vi "SelectorTallestTarget.vi"(0 "Array":T1(array[cluster])) -> (7 "VisionClusterOut":T2={"Position"={"Y"=0.0}, "NoTarget"=TRUE, "Right"=TRUE, "Center"=FALSE, "Left"=TRUE, "TargetCenter"=0.0})   [LabVIEW 2011]
panel:
  out "BetterDistanceV2 - Avg":dbl
  out "BetterDistanceMiddle":dbl
  out "BetterDistanceV1":dbl
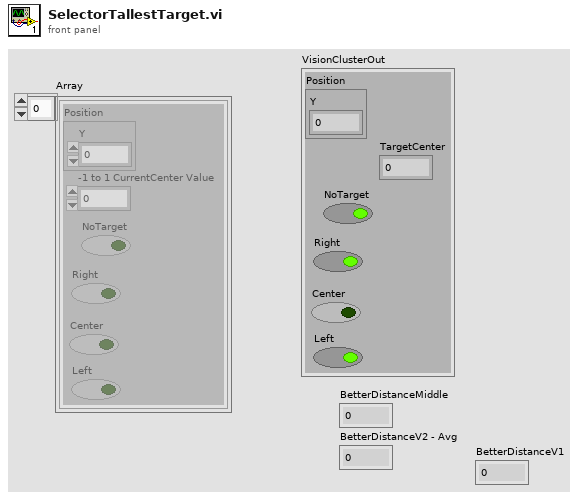
[diagram p1: front panel]
types:
  T1 = cluster{"Position":cluster{"Y":dbl}, "NoTarget":bool, "Right":bool, "Center":bool, "Left":bool, "-1 to 1 CurrentCenter Value":dbl}[]
  T2 = cluster{"Position":cluster{"Y":dbl}, "NoTarget":bool, "Right":bool, "Center":bool, "Left":bool, "TargetCenter":dbl}
  T3 = cluster{"Position":cluster{"X":dbl, "Y":dbl}, "Distance (ft)":dbl, "NoTarget":bool, "Right":bool, "Center":bool, "Left":bool, "TargetCenter":dbl}[]
  T4 = cluster{"Position":cluster{"Y":dbl}, "NoTarget":bool, "Right":bool, "Center":bool, "Left":bool, "-1 to 1 CurrentCenter Value":dbl}
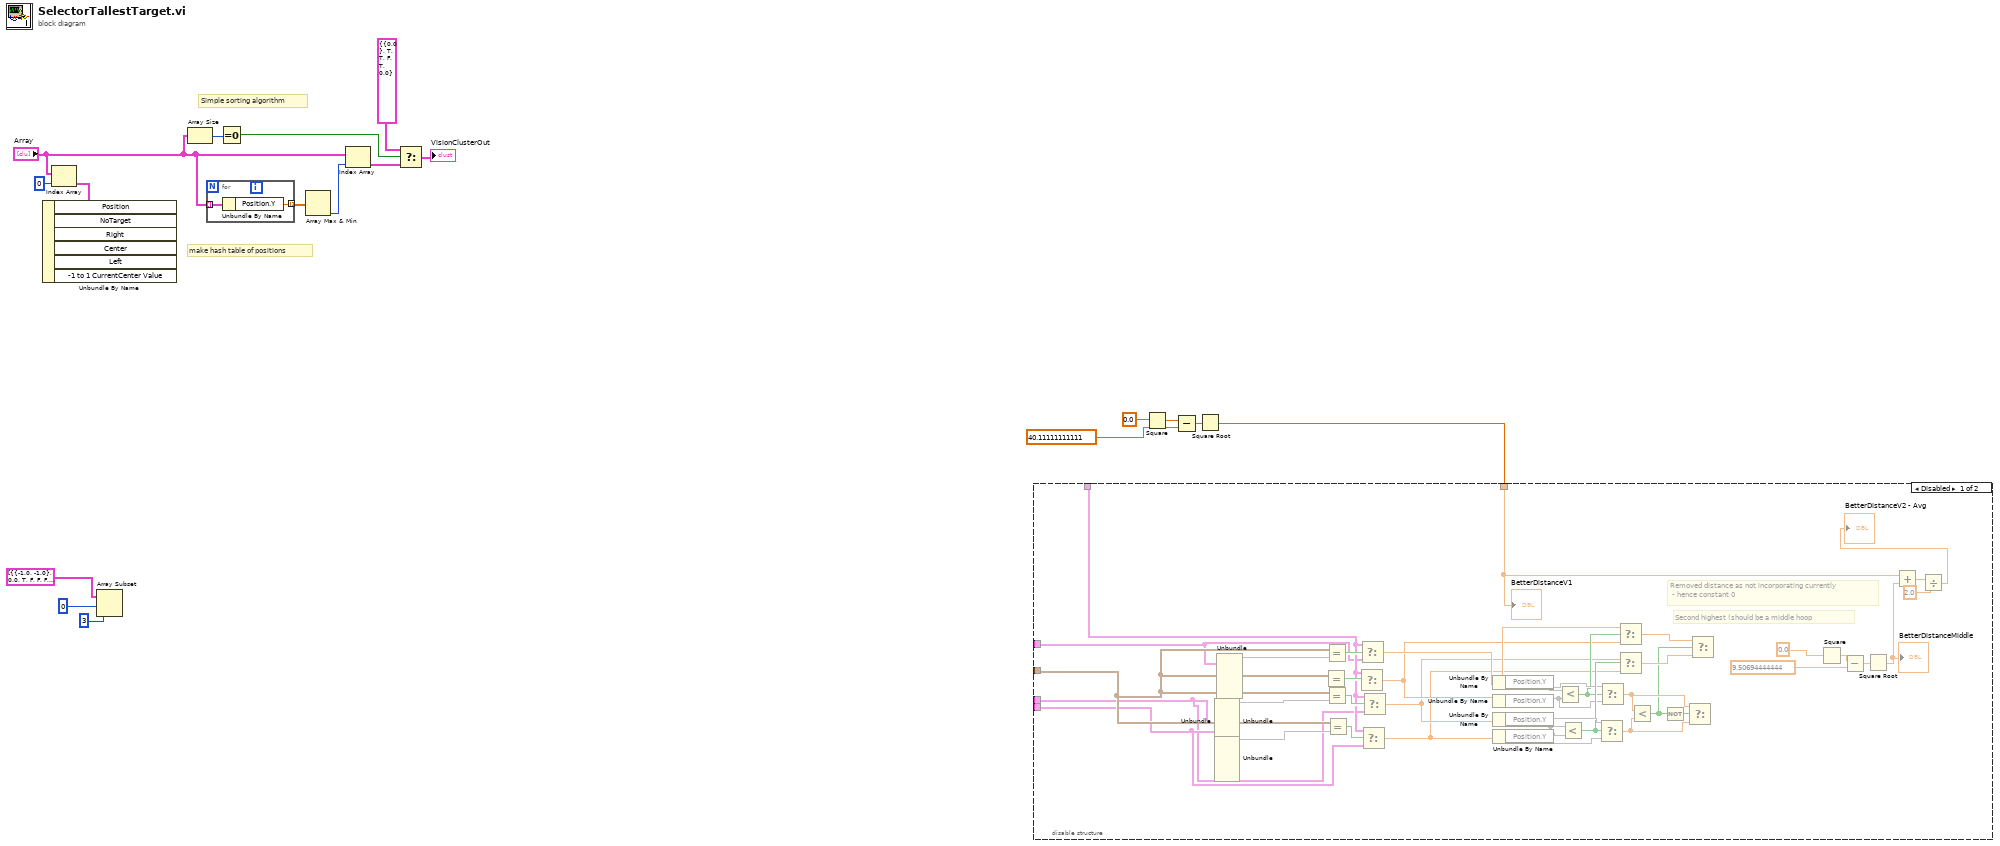
[diagram p0: block diagram]
diagram:
  # "Simple sorting algorithm"
  # "make hash table of positions"
  n1 = Index Array(array="Array", index=0) -> (element=w1:T4)
  n2 = Unbundle By Name(w1) -> ()  [unwired: 6 out]
  n3 = Array Subset(array=T3 [{"Position"={"X"=-1.0, "Y"=-1.0}, "Distance (ft)"=0.0, "NoTarget"=TRUE, "Right"=FALSE, "Center"=FALSE, "Left"=FALSE, "TargetCenter"=0.0}, {"Position"={"X"=0.0, "Y"=0.0}, "Distance (ft)"=16.0, "NoTarget"=FALSE, "Right"=FALSE, "Center"=FALSE, "Left"=TRUE, "TargetCenter"=0.0}, {"Position"={"X"=-0.234375, "Y"=0.5375}, "Distance (ft)"=14.583387907116473, "NoTarget"=FALSE, "Right"=TRUE, "Center"=TRUE, "Left"=FALSE, "TargetCenter"=-0.0234375}, {"Position"={"X"=-0.56875, "Y"=-0.1125}, "Distance (ft)"=16.71013197690429, "NoTarget"=FALSE, "Right"=TRUE, "Center"=FALSE, "Left"=FALSE, "TargetCenter"=-0.190625}] ("Array"), index=0, length=3) -> ()  [unwired: 1 out]
  n4 = Array Size(array="Array") -> (size(s)=w8:i32)
  n5 = for {
    tunnel: "Array" -> [w20] mode=indexing
    tunnel: [w19] -> w10 mode=indexing
    n6 = Unbundle By Name(w20) -> ("Position.Y"=w19:dbl)
  }
  n7 = Equal To 0?(x=w8) -> (x = 0?=w7:bool)
  n8 = Array Max & Min(array=w10) -> (min index (indices)=w9:i32)  [unwired: 3 out]
  n9 = Index Array(array="Array", index=w9) -> (element=w6:T4)
  n10 = Select(t=T2 {"Position"={"Y"=0.0}, "NoTarget"=TRUE, "Right"=TRUE, "Center"=FALSE, "Left"=TRUE, "TargetCenter"=0.0} ("VisionClusterOut"), s=w7, f=w6) -> (s? t:f=→"VisionClusterOut":T4)
  n11 = Square(x=0.0) -> (x^2=w15:dbl)
  n12 = Subtract(x=w15, y=40.11111111111) -> (x-y=w14:dbl)
  n13 = Square Root(x=w14) -> (sqrt(x)=w13:dbl)
  n14 = disable-structure shown="Disabled" {
    disable-tunnel: w13 -> [w39 _]
    disable-tunnel: _ -> [w28 _]
    disable-tunnel: _ -> [w25 _]
    disable-tunnel: _ -> [w24 _]
    disable-tunnel: _ -> [w23 _]
    disable-tunnel: _ -> [w21 _]
    frame Disabled {
      # "Removed distance as not incorporating currently\n - hence constant 0"
      # "Second highest (should be a middle hoop"
      n15 = Unbundle(w21) -> ("Position"=w22)  [unwired: 6 out]
      n16 = Unbundle(w23) -> ()  [unwired: 7 out]
      n17 = Unbundle(w24) -> ("Position"=w27)  [unwired: 6 out]
      n18 = Unbundle(w21) -> ("Position"=w26)  [unwired: 6 out]
      n19 = Equal?(x=w28) -> (x = y?=w56:bool)  [unwired: 1 in]
      n20 = Equal?(x=w28, y=w26) -> (x = y?=w57:bool)
      n21 = Equal?(x=w28, y=w22) -> (x = y?=w55:bool)
      n22 = Equal?(x=w28, y=w27) -> (x = y?=w54:bool)
      n23 = Select(t=w25, s=w56) -> (s? t:f=w32:dbl)  [unwired: 1 in]
      n24 = Select(t=w25, s=w57, f=w21) -> (s? t:f=w33:dbl)
      n25 = Select(t=w25, s=w54, f=w24) -> (s? t:f=w30:dbl)
      n26 = Select(t=w25, s=w55, f=w23) -> (s? t:f=w31:dbl)
      n27 = Unbundle By Name(w33) -> ("Position.Y"=w45)
      n28 = Unbundle By Name(w32) -> ("Position.Y"=w44)
      n29 = Unbundle By Name(w31) -> ("Position.Y"=w50)
      n30 = Unbundle By Name(w30) -> ("Position.Y"=w49)
      n31 = Less?(x=w45, y=w44) -> (x < y?=w43:bool)
      n32 = Less?(x=w50, y=w49) -> (x < y?=w46:bool)
      n33 = Select(t=w50, s=w46, f=w49) -> (s? t:f=w52:dbl)
      n34 = Select(t=w45, s=w43, f=w44) -> (s? t:f=w51:dbl)
      n35 = Select(t=w33, s=w43, f=w32) -> (s? t:f=w47:dbl)
      n36 = Select(t=w31, s=w46, f=w30) -> (s? t:f=w48:dbl)
      n37 = Less?(x=w51, y=w52) -> (x < y?=w34:bool)
      n38 = Not(x=w34) -> (.not. x?=w53:bool)
      n39 = Select(t=w51, s=w53, f=w52) -> ()  [unwired: 1 out]
      n40 = Select(t=w47, s=w34, f=w48) -> ()  [unwired: 1 out]
      n41 = Square(x=0.0) -> (x^2=w41:dbl)
      n42 = Subtract(x=w41, y=9.50694444444) -> (x-y=w42:dbl)
      n43 = Square Root(x=w42) -> (sqrt(x)=w38:dbl)
      "BetterDistanceMiddle" <- w38
      n44 = Add(x=w39, y=w38) -> (x+y=w37:dbl)
      n45 = Divide(x=w37, y=2.0) -> (x/y=→"BetterDistanceV2 - Avg":dbl)
      "BetterDistanceV1" <- w39
    }
    frame Enabled {
    }
  }
